vi "Destroy.vi"(0 "reference":refnum<class "StateDiagramGraph.lvclass">, 5 "error in (no error)":errorcluster) -> (19 "error out":errorcluster)   [LabVIEW 2014, in "StateDiagramGraph.lvclass"]
doc: "Destroys a StateDiagramGraph object created with a StateDiagramGraph constructor VI.\n\n[GOOP 2.1]"
uses:
  <resource>/Framework/Providers/Open_GDS/UML/StateDiagramGraph_class/StateDiagramGraph.lvclass
  <resource>/Framework/Providers/Open_GDS/UML/Graph_class/Graph.lvclass
panel:
  out "reference out":refnum<class "StateDiagramGraph.lvclass">
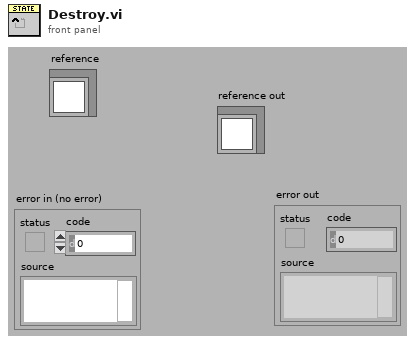
[diagram p1: front panel]
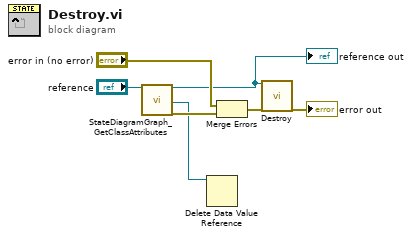
[diagram p0: block diagram]
diagram:
  n1 = call <resource>:"StateDiagramGraph_GetClassAttributes.vi"("reference in"="reference") -> ("reference out"=w3:refnum<class "StateDiagramGraph.lvclass">, "Class attribute Reference"=w1:refnum<data-value>, "error out"=w4:errorcluster)  [unwired: 1 in, 15 out]
  "reference out" <- w3
  n2 = Delete Data Value Reference(data value reference=w1) -> ()  [unwired: 1 in, 2 out]
  n3 = Merge Errors("error in (no error)", w4) -> (w2:errorcluster)
  n4 = call-parent "Destroy.vi"("reference"=w3, "error in (no error)"=w2) -> ("error out"=→"error out":errorcluster)  [unwired: 17 in]
